vi "Run.vi"(7 "Team Index":i32, 8 "Column":i32, 9 "Row":i32, 10 "View":i32[](array[numeric]) caption="View (Team Index, -1: empty)", 11 "AndrewF In":refnum<class "AndrewF.lvclass">) -> (0 "Replicated":refnum<class "Square.lvclass">, 1 "Direction":T1, 2 "Action":T2, 3 "AndrewF Out":refnum<class "Square.lvclass">)   [LabVIEW 2016, in "AndrewF.lvclass"]
uses:
  AndrewF.lvclass
  C:/Users/Events/Desktop/SquareBattle/Square/Square.lvclass
  Square/Square.lvclass
  Type Defs/Action Enum.ctl
  Type Defs/Direction Enum.ctl
  AndrewF.lvclass/AndrewF.ctl
  Common/Common.lvlib
  Type Defs/SB Type Defs.lvlib
panel:
  # "NW\nN\nNE\nE\nSE\nS\nSW\nW"
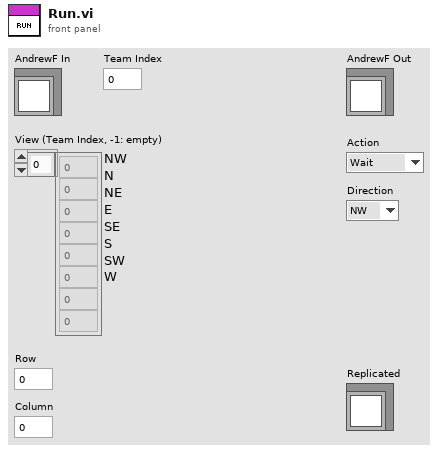
[diagram p1: front panel]
types:
  T1 = typedef "SB Type Defs.lvlib/Direction Enum.ctl" = enum16{"NW", "N", "NE", "E", "SE", "S", "SW", "W"}
  T2 = typedef "SB Type Defs.lvlib/Action Enum.ctl" = enum16{"Wait", "Move", "Attack", "Replicate"}
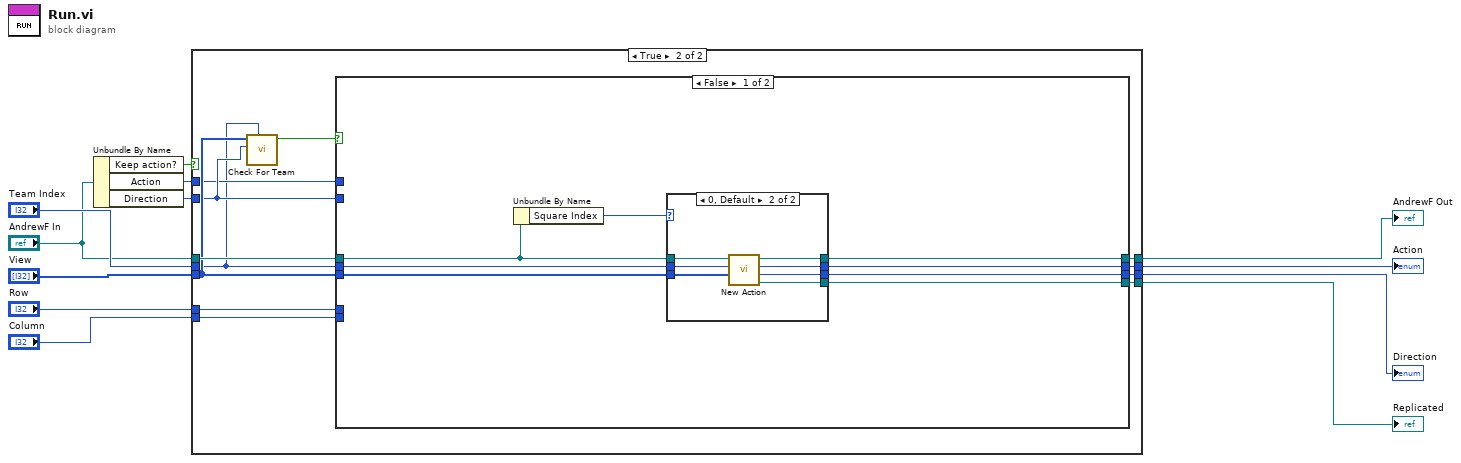
[diagram p0: block diagram]
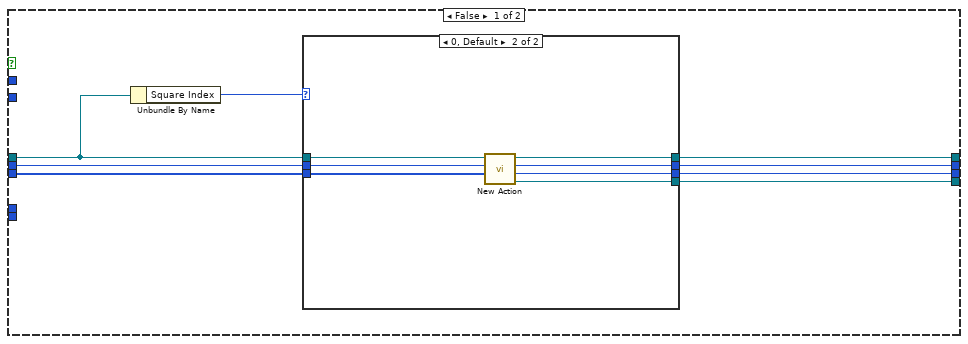
[diagram p2: hidden frame]
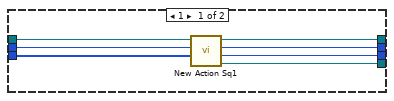
[diagram p3: hidden frame]
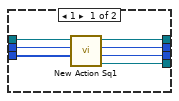
[diagram p4: hidden frame]
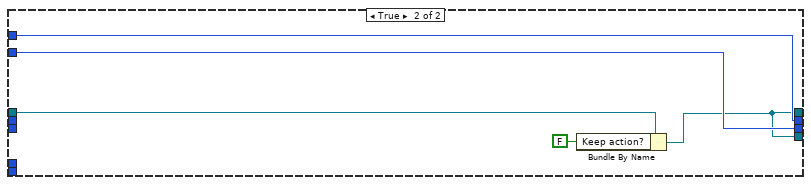
[diagram p5: hidden frame]
diagram:
  n1 = Unbundle By Name("AndrewF In") -> ("Keep action?"=w2:bool, "Action"=w1:T2, "Direction"=w6:T1)
  n2 = case shown="True" w2 {
    tunnel: [w15 w46] -> w12
    tunnel: [w18 w45] -> w11
    tunnel: "Column" -> [_ w44]
    tunnel: "Row" -> [_ w43]
    tunnel: "Team Index" -> [w20 w35]
    tunnel: "AndrewF In" -> [w14 w42]
    tunnel: w6 -> [_ w38]
    tunnel: [w17 w41] -> w5
    tunnel: "View" -> [w19 w39]
    tunnel: [w16 w40] -> w3
    tunnel: w1 -> [_ w36]
    frame False {
      n3 = Unbundle By Name(w14) -> ("Square Index"=w13:i32)
      n4 = case shown="0, Default" w13 {
        tunnel: w14 -> [w27 w34]
        tunnel: w20 -> [w26 w33]
        tunnel: w19 -> [w25 w32]
        tunnel: [w24 w31] -> w18
        tunnel: [w23 w30] -> w17
        tunnel: [w22 w29] -> w16
        tunnel: [w21 w28] -> w15
        frame 1 {
          n5 = call-dynamic "New Action Sq1.vi"("View"=w25, "Team Index"=w26, "AndrewF in"=w27) -> ("Replicated"=w21:refnum<class "Square.lvclass">, "Direction"=w22:T1, "Action"=w23:T2, "AndrewF out"=w24:refnum<class "AndrewF.lvclass">)  [unwired: 5 in]
        }
        frame 0, Default {
          n6 = call-dynamic "New Action.vi"("View"=w32, "Team Index"=w33, "AndrewF in"=w34) -> ("Replicated"=w28:refnum<class "Square.lvclass">, "Direction"=w29:T1, "Action"=w30:T2, "AndrewF out"=w31:refnum<class "AndrewF.lvclass">)  [unwired: 5 in]
        }
      }
    }
    frame True {
      n7 = call "Check For Team.vi"("Team Index"=w35, "Direction"=w38, "Map"=w39) -> ("Clear?"=w37:bool)  [unwired: 8 in]
      n8 = case shown="False" w37 {
        tunnel: [w49 w69] -> w46
        tunnel: [w50 w69] -> w45
        tunnel: w44 -> [_ _]
        tunnel: w43 -> [_ _]
        tunnel: w35 -> [w54 _]
        tunnel: w42 -> [w48 w70]
        tunnel: [w51 w73] -> w41
        tunnel: [w52 w72] -> w40
        tunnel: w39 -> [w53 _]
        tunnel: w38 -> [_ w72]
        tunnel: w36 -> [_ w73]
        frame False {
          n9 = Unbundle By Name(w48) -> ("Square Index"=w47:i32)
          n10 = case shown="0, Default" w47 {
            tunnel: w54 -> [w61 w68]
            tunnel: w53 -> [w60 w67]
            tunnel: [w59 w66] -> w52
            tunnel: [w58 w65] -> w51
            tunnel: [w57 w64] -> w50
            tunnel: [w56 w63] -> w49
            tunnel: w48 -> [w55 w62]
            frame 1 {
              n11 = call-dynamic "New Action Sq1.vi"("View"=w60, "Team Index"=w61, "AndrewF in"=w55) -> ("Replicated"=w56:refnum<class "Square.lvclass">, "Direction"=w59:T1, "Action"=w58:T2, "AndrewF out"=w57:refnum<class "AndrewF.lvclass">)  [unwired: 5 in]
            }
            frame 0, Default {
              n12 = call-dynamic "New Action.vi"("View"=w67, "Team Index"=w68, "AndrewF in"=w62) -> ("Replicated"=w63:refnum<class "Square.lvclass">, "Direction"=w66:T1, "Action"=w65:T2, "AndrewF out"=w64:refnum<class "AndrewF.lvclass">)  [unwired: 5 in]
            }
          }
        }
        frame True {
          n13 = Bundle By Name(cluster=w70, "Keep action?"=FALSE) -> (w69:refnum<class "AndrewF.lvclass">)
        }
      }
    }
  }
  "AndrewF Out" <- w11
  "Action" <- w5
  "Direction" <- w3
  "Replicated" <- w12
